vi "Transmit Lockin Data.vi"(8 "error in (no error)":errorcluster, 10 "Data":dbl[](array[numeric]), 11 "RP Transceiver in":refnum<class "RP Transceiver.lvclass">) -> (0 "error out":errorcluster, 2 "First phase word":i32, 3 "RP Transceiver out":refnum<class "RP Transceiver.lvclass">)   [LabVIEW 2015, in "RP Transceiver.lvclass"]
uses:
  RP Transceiver.lvclass
  RP Transceiver.lvclass/RP Transceiver.ctl
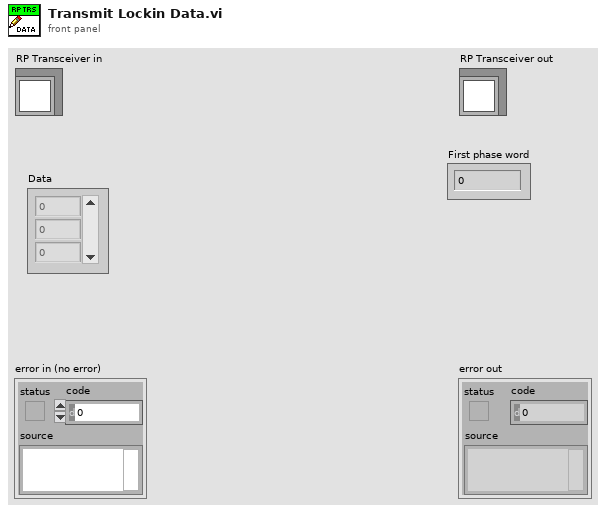
[diagram p1: front panel]
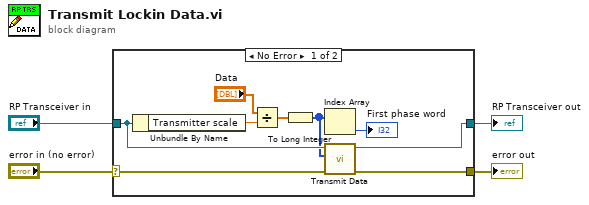
[diagram p0: block diagram]
diagram:
  n1 = case shown="No Error" "error in (no error)" {
    selector: "error in (no error)" -> [w8 w15]
    tunnel: [w7 w15] -> w3
    tunnel: [w13 w14] -> w1
    tunnel: "RP Transceiver in" -> [w12 w14]
    frame No Error {
      n2 = Unbundle By Name(w12) -> ("Transmitter scale"=w10:dbl)
      n3 = Divide(x="Data", y=w10) -> (x/y=w9:dbl[])
      n4 = To Long Integer(number=w9) -> (32bit integer=w6:i32[])
      n5 = Index Array(array=w6) -> (element=→"First phase word":i32)  [unwired: 1 in]
      n6 = call-dynamic "Transmit Data.vi"("error in (no error)"=w8, "Data"=w6, "RP Transceiver in"=w12) -> ("error out"=w7:errorcluster, "RP Transceiver out"=w13:refnum<class "RP Transceiver.lvclass">)  [unwired: 7 in]
    }
    frame Error {
    }
  }
  "error out" <- w3
  "RP Transceiver out" <- w1
